vi "GetPlayerName.vi"(8 "error in (no error)":errorcluster, 11 "Player in":refnum<class "Player.lvclass">) -> (0 "error out":errorcluster, 2 "PlayerName":string, 3 "Player out":refnum<class "Player.lvclass">)   [LabVIEW 2015, in "TronviewGame.lvlib" / "Player.lvclass"]
uses:
  Player.lvclass
  Player.lvclass/Player.ctl
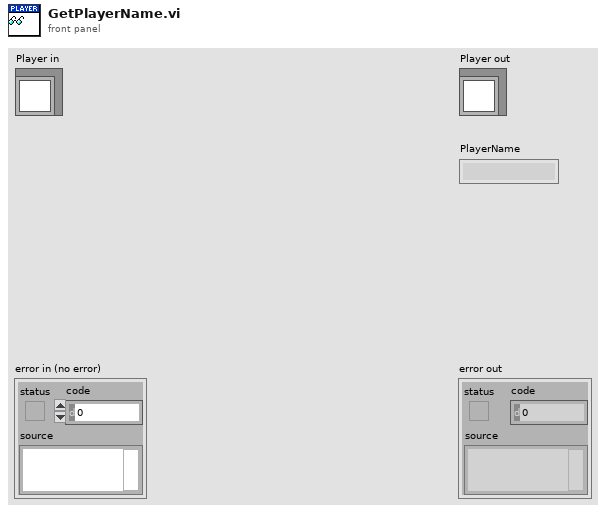
[diagram p1: front panel]
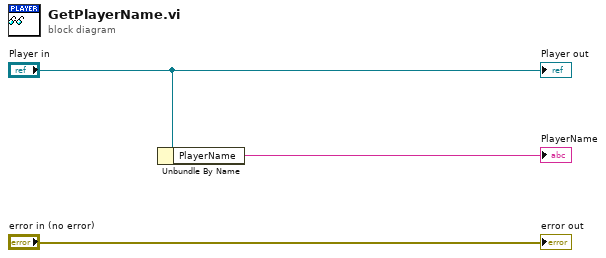
[diagram p0: block diagram]
diagram:
  n1 = Unbundle By Name("Player in") -> ("PlayerName"=→"PlayerName":string)
  "error out" <- "error in (no error)"
  "Player out" <- "Player in"
